vi "Install Set 1.0.vi"(7 "Restart Automatically (T)":bool=TRUE, 8 "error in (no error)":errorcluster, 9 "Add-on IDs":string[](array[string]), 10 "Software Set ID":string, 11 "Session in":refnum<k21>) -> (0 "error out":errorcluster, 1 "Broken Dependencies":T1[](array[typedef]), 3 "Session out":refnum<k21>)   [LabVIEW 2014, in "nisyscfg.lvlib"]
uses:
  nisyscfg.lvlib
  Broken Dependency.ctl
  Software.ctl
  Software 1.2.ctl
  Component Type.ctl
  Install Set.vi
panel:
  # "This cluster is deprecated.\nUse Broken Dependency 1.2.ctl."
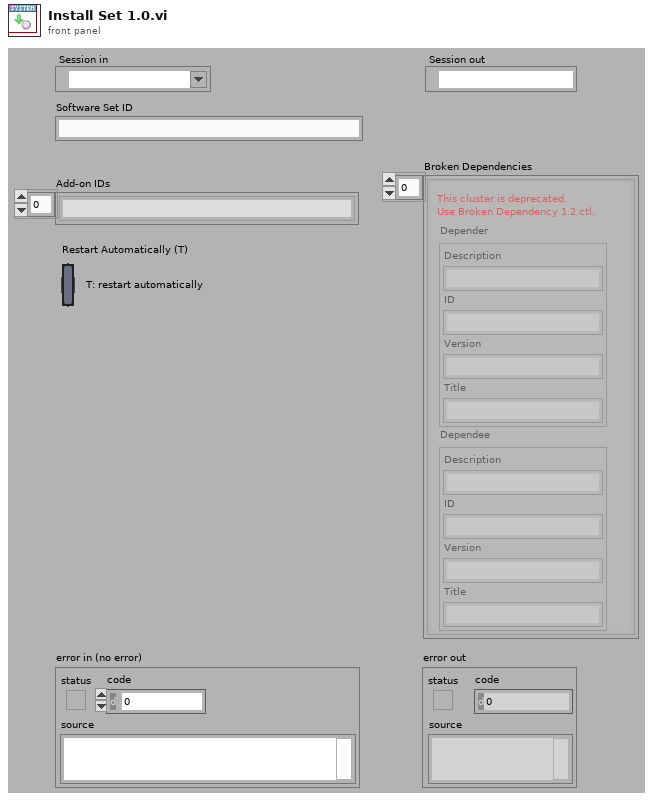
[diagram p1: front panel]
types:
  T1 = typedef "nisyscfg.lvlib/Broken Dependency.ctl" = cluster{"Depender":T2, "Dependee":T2}
  T2 = typedef "nisyscfg.lvlib/Software.ctl" = cluster{"Description":string, "ID":string, "Version":string, "Title":string}
  T3 = typedef "nisyscfg.lvlib/Software 1.2.ctl" = cluster{"title":string, "description":string, "ID":string, "version":string, "component type":T4}
  T4 = typedef "nisyscfg.lvlib/Component Type.ctl" = u32
  T5 = typedef "nisyscfg.lvlib/Broken Dependency 1.2.ctl" = cluster{"depender":T3, "dependee":T3}
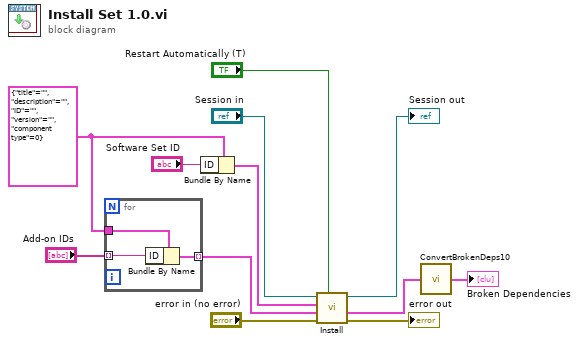
[diagram p0: block diagram]
diagram:
  w1 = T3 {"title"="", "description"="", "ID"="", "version"="", "component type"=0} ("software")
  n1 = for {
    tunnel: w1 -> [w15]
    tunnel: "Add-on IDs" -> [w14] mode=indexing
    tunnel: [w13] -> w4 mode=indexing
    n2 = Bundle By Name(cluster=w15, "ID"=w14) -> (w13:T3)
  }
  n3 = Bundle By Name(cluster=w1, "ID"="Software Set ID") -> (w3:T3)
  n4 = call-poly "Install.vi"("Restart Automatically (T)"="Restart Automatically (T)", "error in (no error)"="error in (no error)", "Add-ons to Install"=w4, "Software Set"=w3, "Session in"="Session in") -> ("error out"=→"error out":errorcluster, "Broken Dependencies"=w6:T5[], "Session out"=→"Session out":refnum<k21>)  [unwired: 4 in]
  n5 = call "ConvertBrokenDeps10.vi"("dependencies 1.2"=w6) -> ("dependencies 1.0"=→"Broken Dependencies":T1[])
